vi "Exit.vi"(8 "error in (no error)":errorcluster, 11 "Old State":refnum<class "State3.lvclass">) -> (0 "error out":errorcluster, 3 "New State":refnum<class "State3.lvclass">)   [LabVIEW 2025, in "Demo_States.lvlib" / "State3.lvclass"]
doc: "This is an abstract method. Override this method to define the behavior when you leave the state."
uses:
  State3.lvclass
  State3.lvclass/State3.ctl
  Demo_States/Demo_States.lvclass
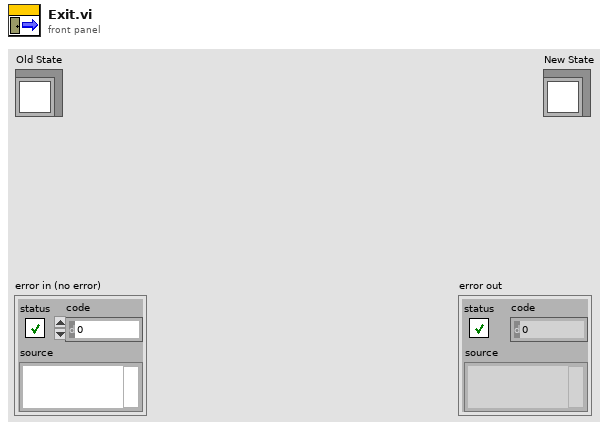
[diagram p1: front panel]
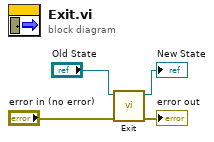
[diagram p0: block diagram]
diagram:
  n1 = call-parent "Exit.vi"("error in (no error)"="error in (no error)", "Old State"="Old State") -> ("error out"=→"error out":errorcluster, "New State"=→"New State":refnum<class "State3.lvclass">)  [unwired: 8 in]
